vi "meTEC_Read_ID 4010_Object Temperature_Lower Error Threshold.vi"(6 "Instance (1)":u8=1, 8 "error in (no error)":errorcluster, 9 "TEC Configuration_IN":T1={"VISA resource name"="", "Device Address"=2}, 10 "Sequence No.":u16=5552) -> (0 "error out":errorcluster, 1 "TEC Configuration_OUT":T1={"VISA resource name"="", "Device Address"=2}, 3 "Object Temperature_Lower Error Threshold [°C] (ID 4010)":dbl format="%#.3f")   [LabVIEW 2010]
uses:
  TypeDefs/meTEC_Configuration.ctl
panel:
  # "--- Inputs ---"
  # "--- Outputs ---"
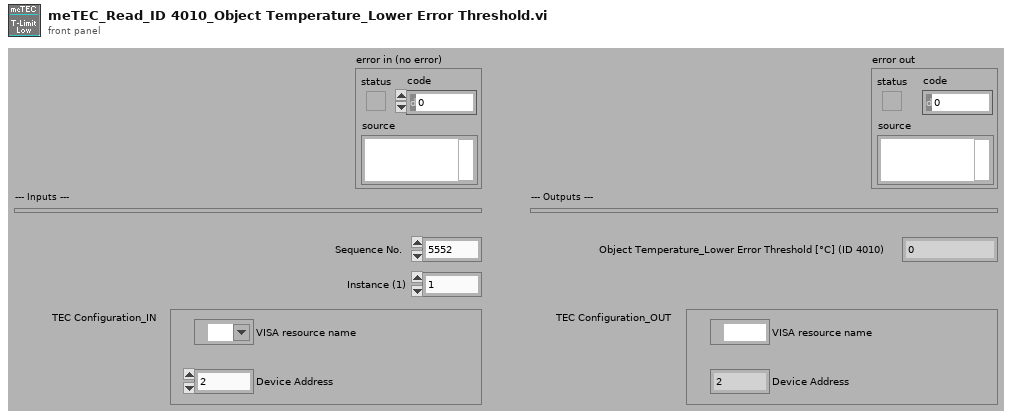
[diagram p1: front panel]
types:
  T1 = typedef "meTEC_Configuration.ctl" = cluster{"VISA resource name":refnum<visa-resource-name>, "Device Address":u16}
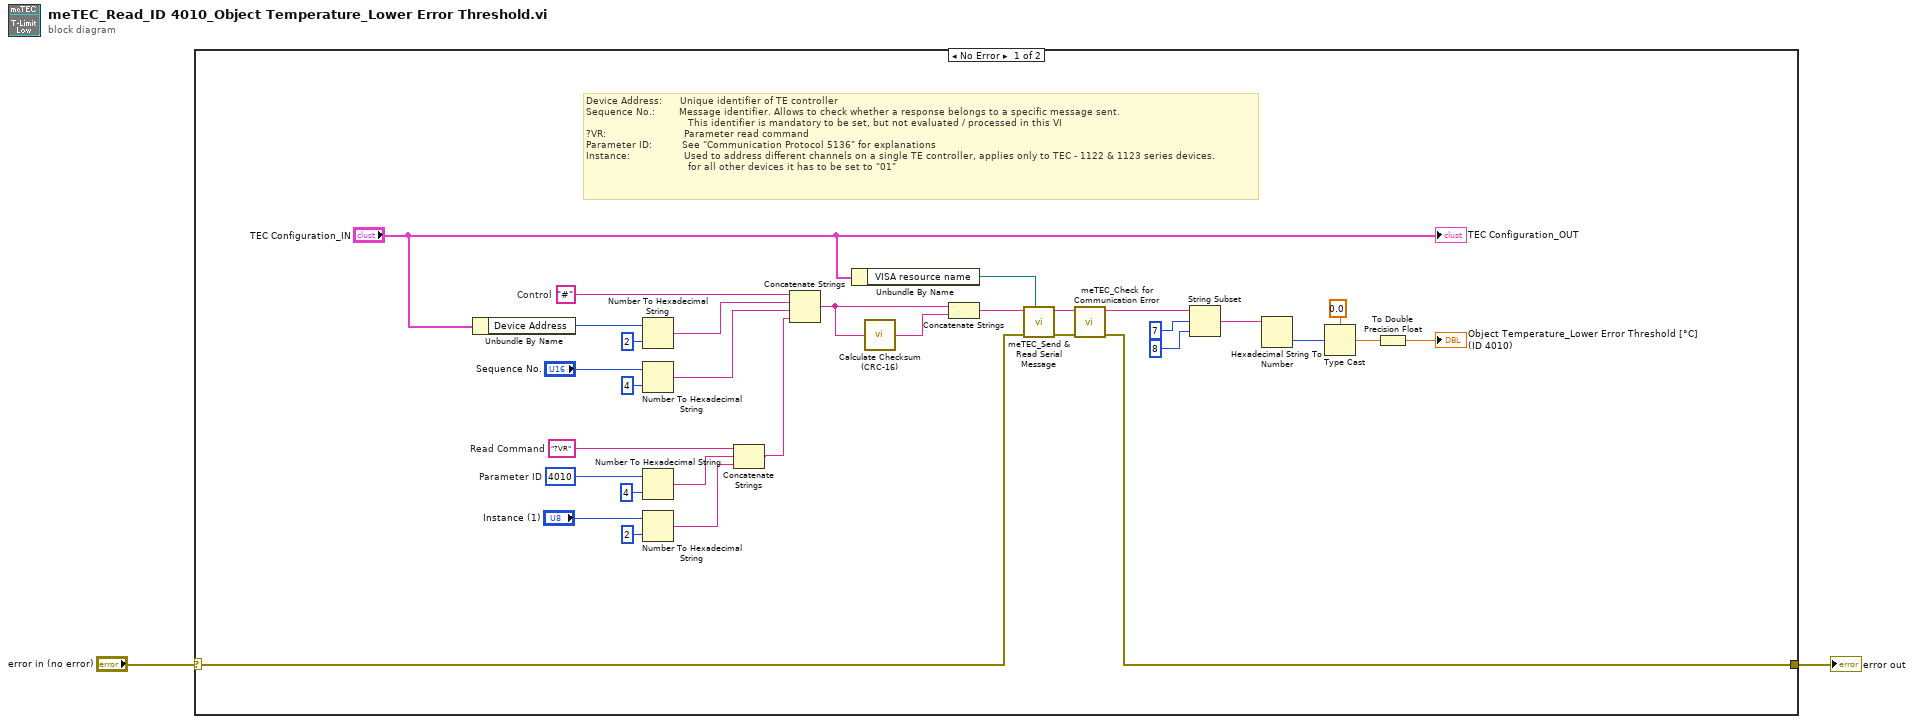
[diagram p0: block diagram]
diagram:
  n1 = case shown="No Error" "error in (no error)" {
    selector: "error in (no error)" -> [w13 w35]
    tunnel: [w5 w35] -> w2
    frame No Error {
      w23 = 4010  # Parameter ID
      w24 = "?VR"  # Read Command
      w32 = "#"  # Control
      # "Device Address:      Unique identifier of TE controller\nSequence No.:        Message identifier. Allows to check whether a response belongs to a specific message sent.\n                                  This identifier is mandatory to be set, but not evaluated / processed in this VI\n?VR:                          Parameter read command\nParameter ID:          See \"Communication Protocol 5136\" for explanations\nInstance:                  Used to address different channels on a single TE controller, applies only to TEC - 1122 & 1123 series devices.\n                                  for all other devices it has to be set to \"01\""
      n2 = Unbundle By Name("TEC Configuration_IN") -> ("Device Address"=w8:u16)
      n3 = Number To Hexadecimal String(1:i16 2 ("width (-)"), 2:w8) -> (0:w27:string)
      n4 = Number To Hexadecimal String(1:i16 4 ("width (-)"), 2:"Sequence No.") -> (0:w31:string)
      n5 = Number To Hexadecimal String(1:i16 4 ("width (-)"), 2:w23) -> (0:w25:string)
      n6 = Number To Hexadecimal String(1:i16 2 ("width (-)"), 2:"Instance (1)") -> (0:w10:string)
      n7 = Concatenate Strings(w24, w25, w10) -> (w21:string)
      n8 = Concatenate Strings(w32, w27, w31, w21) -> (w30:string)
      n9 = Unbundle By Name("TEC Configuration_IN") -> ("VISA resource name"=w9:refnum<visa-resource-name>)
      n10 = call "Calculate Checksum (CRC-16).vi"("Message"=w30) -> ("CRC [String]"=w29:string)  [unwired: 1 in]
      n11 = Concatenate Strings(w30, w29) -> (w26:string)
      n12 = call "meTEC_Send & Read Serial Message.vi"("VISA resource name"=w9, "error in (no error)"=w13, "Serial Message"=w26) -> ("error out"=w12:errorcluster, "Serial Message_Read"=w4:string)  [unwired: 7 in]
      n13 = call "meTEC_Check for Communication Error.vi"("error in (no error)"=w12, "Serial Message_IN"=w4) -> ("error out"=w5:errorcluster, "Serial Message_OUT"=w3:string)  [unwired: 8 in]
      n14 = String Subset(string=w3, offset (0)=7, length (rest)=8 ("length (rest)")) -> (substring=w18:string)
      n15 = Hexadecimal String To Number(string=w18) -> (number=w15:u32)  [unwired: 2 in, 1 out]
      n16 = Type Cast(type=sgl 0.0, x=w15) -> (*(type *) &x=w14:sgl)
      n17 = To Double Precision Float(number=w14) -> (double precision float=→"Object Temperature_Lower Error Threshold [°C] (ID 4010)":dbl)
      "TEC Configuration_OUT" <- "TEC Configuration_IN"
    }
    frame Error {
    }
  }
  "error out" <- w2
